vi "test Wrapper VIs.vi"(8 "error in (no error)":errorcluster, 11 "TestCase in":refnum<class "Scan Engine Unit Tests.lvclass">) -> (0 "error out":errorcluster, 3 "TestCase out":refnum<class "Scan Engine Unit Tests.lvclass">)   [LabVIEW 2019, in "Scan Engine Unit Tests.lvclass"]
uses:
  Scan Engine Unit Tests.lvclass
  <vilib>/addons/_JKI Toolkits/VI Tester/TestCase.llb/TestCase.lvclass
  C:/Program Files (x86)/National Instruments/LabVIEW 2019/vi.lib/addons/_JKI Toolkits/VI Tester/TestCase.llb/TestCase.lvclass
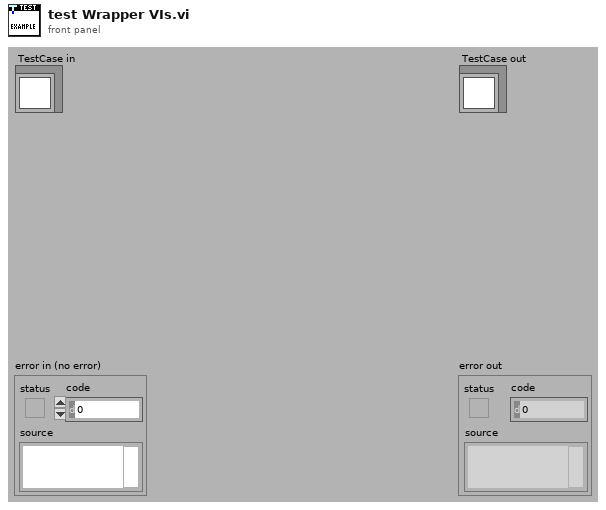
[diagram p1: front panel]
types:
  T1 = enum32{"Bad", "Idle", "Run top level", "Running"}
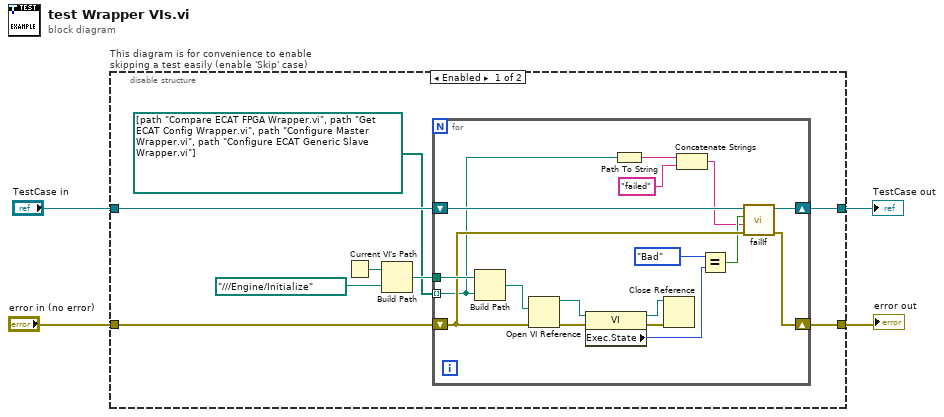
[diagram p0: block diagram]
diagram:
  n1 = disable-structure "This diagram is for convenience to enable skipping a test easily (enable 'Skip' case)" shown="Enabled" {
    disable-tunnel: "TestCase in" -> [w12 w33]
    disable-tunnel: [w7 w31] -> w1
    disable-tunnel: [w8 w32] -> w3
    disable-tunnel: "error in (no error)" -> [w9 w30]
    frame Enabled {
      n2 = Current VI's Path() -> (path=w11:path)
      n3 = Build Path(base path=w11, name or relative path=path "../../../Engine/Initialize" ("vi path")) -> (appended path=w6:path)
      n4 = for {
        tunnel: w6 -> [w27]
        shift-right: [w22] -> w7
        shift-left: w12 -> [w29]
        shift-right: [w23] -> w8
        shift-left: w9 -> [w26]
        tunnel: path[] [path "Compare ECAT FPGA Wrapper.vi", path "Get ECAT Config Wrapper.vi", path "Configure Master Wrapper.vi", path "Configure ECAT Generic Slave Wrapper.vi"] -> [w17] mode=indexing
        n5 = Build Path(base path=w27, name or relative path=w17) -> (appended path=w28:path)
        n6 = Open VI Reference(vi path=w28, error in (no error)=w26) -> (vi reference=w24:refnum<vi>, error out=w25:errorcluster)  [unwired: 4 in]
        n7 = property class="VI"(reference=w24, error in=w25) -> (reference out=w20:refnum<vi>, error out=w21:errorcluster, "Exec.State"=w15:T1)
        n8 = Path To String(path=w17) -> (string=w18:string)
        n9 = Close Reference(reference=w20, error in (no error)=w21) -> ()  [unwired: 1 out]
        n10 = Concatenate Strings(w18, "failed" ("custom report message (\"\")")) -> (w13:string)
        n11 = Equal?(x=T1."Bad" ("Execution:State"), y=w15) -> (x = y?=w14:bool)
        n12 = call-dynamic "failIf.vi"("error in (no error)"=w26, "message (\"\")"=w13, "fail"=w14, "TestCase in"=w29) -> ("error out"=w23:errorcluster, "TestCase out"=w22:refnum<class "Scan Engine Unit Tests.lvclass">)  [unwired: 6 in]
      }
    }
    frame Disabled {
      # "skip test result while test is under development"
      n13 = call <vilib>:"skip.vi"("error in (no error)"=w30, "TestCase in"=w33) -> ("error out"=w32:errorcluster, "TestCase out"=w31:refnum<class "Scan Engine Unit Tests.lvclass">)  [unwired: 8 in]
    }
  }
  "error out" <- w3
  "TestCase out" <- w1
